vi "myRIO v1.0 Build MUX Configuration AO.vi"(11 "AO Channels List":T4) -> (3 "Channel Reservation Info":T1)   [LabVIEW 2021]
uses:
  <vilib>/myRIO/Common/Instrument Driver Framework/myRIO v1.0/AO/typedefs/AO Channels List.ctl
  <vilib>/myRIO/Common/Instrument Driver Framework/myRIO v1.0/AO/typedefs/AO Channels Enum.ctl
  <vilib>/myRIO/Common/Instrument Driver Framework/myRIO v1.0/Resource Manager/typedefs/myRIO v1.0 Channel Reservation List.ctl
  <vilib>/myRIO/Common/Instrument Driver Framework/myRIO v1.0/Resource Manager/typedefs/myRIO v1.0 Channel Reservation Info.ctl
  <vilib>/myRIO/Common/Instrument Driver Framework/myRIO v1.0/Resource Manager/typedefs/myRIO v1.0 Connector List.ctl
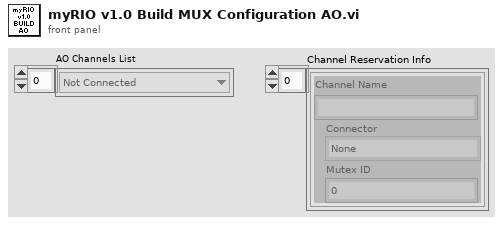
[diagram p1: front panel]
types:
  T1 = typedef "myRIO v1.0 Channel Reservation List.ctl" = T2[]
  T2 = typedef "myRIO v1.0 Channel Reservation Info.ctl" = cluster{"Channel Name":string, "Connector":T3, "Mutex ID":i32}
  T3 = typedef "myRIO v1.0 Connector List.ctl" = enum32{"None", "ConnectorA", "ConnectorB", "ConnectorC"}
  T4 = typedef "AO Channels List.ctl" = T5[]
  T5 = typedef "AO Channels Enum.ctl" = enum16{"Not Connected", "AudioOut/Left", "AudioOut/Right", "C/AO0", "C/AO1", "A/AO0", "A/AO1", "B/AO0", "B/AO1"}
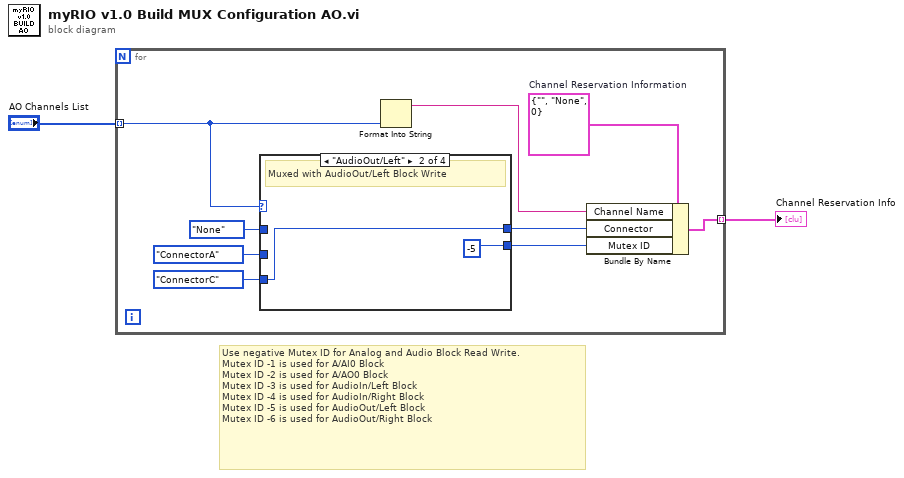
[diagram p0: block diagram]
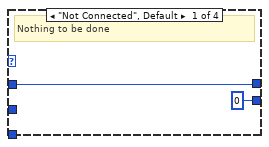
[diagram p2: hidden frame]
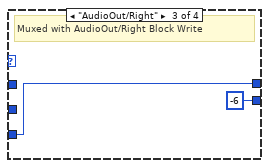
[diagram p3: hidden frame]
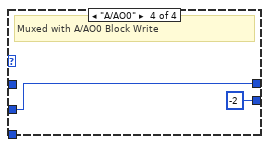
[diagram p4: hidden frame]
diagram:
  # "Use negative Mutex ID for Analog and Audio Block Read Write.\nMutex ID -1 is used for A/AI0 Block\nMutex ID -2 is used for A/AO0 Block\nMutex ID -3 is used for AudioIn/Left Block\nMutex ID -4 is used for AudioIn/Right Block\nMutex ID -5 is used for AudioOut/Left Block\nMutex ID -6 is used for AudioOut/Right Block"
  n1 = for {
    tunnel: "AO Channels List" -> [w8] mode=indexing
    tunnel: [w9] -> w1 mode=indexing
    w11 = T2 {"Channel Name"="", "Connector"=enum."None", "Mutex ID"=0}  # Channel Reservation Information
    n2 = case shown="\"AudioOut/Left\"" w8 {
      tunnel: [w12 w14 w17 w18] -> w7
      tunnel: [0 ("Bit") -5 ("Bit") -6 ("Bit") -2 ("Bit")] -> w6
      tunnel: myRIO_v1.0_Connector_List."ConnectorC" ("Connector") -> [_ w14 w17 _]
      tunnel: myRIO_v1.0_Connector_List."None" ("Connector") -> [w12 _ _ _]
      tunnel: myRIO_v1.0_Connector_List."ConnectorA" ("Connector") -> [_ _ _ w18]
      frame "Not Connected", Default {
        # "Nothing to be done"
      }
      frame "AudioOut/Left" {
        # "Muxed with AudioOut/Left Block Write"
      }
      frame "AudioOut/Right" {
        # "Muxed with AudioOut/Right Block Write"
      }
      frame "A/AO0" {
        # "Muxed with A/AO0 Block Write"
      }
    }
    n3 = Format Into String(w8) -> (resulting string=w10:string)  [unwired: 3 in, 1 out]
    n4 = Bundle By Name(cluster=w11, "Channel Name"=w10, "Connector"=w7, "Mutex ID"=w6) -> (w9:T2)
  }
  "Channel Reservation Info" <- w1
